vi "S2DS_External control parameters (SubVI).vi"(11 "Array in":i32[](array[numeric])) -> (3 "Array out":i32[](array[numeric]))   [LabVIEW 2025]
panel:
  in  "Check interval (ms)":i32
  in  "Timeout (s)":i32
  in  "Cancel":bool
  in  "OK":bool
  # "Set parameters for checking \nexternal controller's response..."
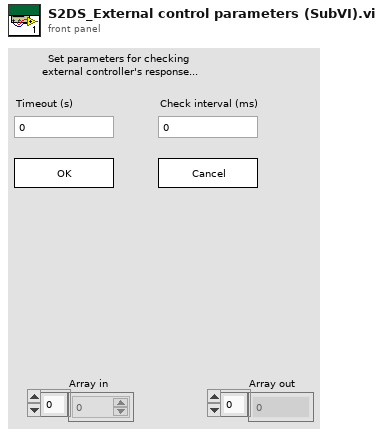
[diagram p1: front panel]
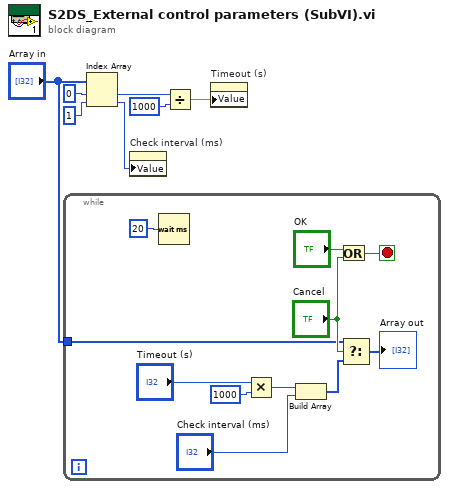
[diagram p0: block diagram]
diagram:
  n1 = while {
    tunnel: "Array in" -> [w11]
    stop <- w17 stop-if-true
    n2 = Wait (ms)(milliseconds to wait=u32 20) -> ()  [unwired: 1 out]
    n3 = Multiply(x="Timeout (s)", y=1000) -> (x*y=w8:i32)
    n4 = Build Array(w8, "Check interval (ms)") -> (w14:i32[])
    n5 = Or(x="OK", y="Cancel") -> (x .or. y?=w17:bool)
    n6 = Select(t=w11, s="Cancel", f=w14) -> (s? t:f=→"Array out":i32[])
  }
  n7 = Index Array(array="Array in", index #1=0 ("index"), index #2=1 ("index")) -> (element #1=w3:i32, element #2=w4:i32)
  n8 = property on="Check interval (ms)" class="DigNum (strict)"("Value"=w4) -> ()  [unwired: 2 in, 2 out]
  n9 = Divide(x=w3, y=1000) -> (x/y=w1:dbl)
  n10 = property on="Timeout (s)" class="DigNum (strict)"("Value"=w1) -> ()  [unwired: 2 in, 2 out]
